vi "arm pid.vi"(2 "Setpoint":dbl, 3 "Autotune?":bool) -> (0 "Output":dbl)   [LabVIEW 2013]
uses:
  typedefs/fg_typedef.ctl
  typedefs/DevRef Type.ctl
  <vilib>/addons/control/pid/pid.llb/PID (DBL).vi
  <vilib>/addons/control/pid/NI_PID_autopid.lvlib
  <vilib>/addons/control/pid/NI_PID_pid.lvlib
panel:
  in  "autotuning parameters":T1={"controller type"=1, "relay cycles"=3, "relay amplitude"=1.0, "control specification"=2, "PV noise level"=0.1} {"controller type" items=["PID", "PI", "P"]; "control specification" items=["normal", "fast", "slow"]}
  # "Things needing Tuning"
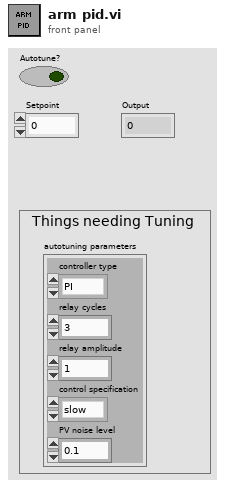
[diagram p1: front panel]
types:
  T1 = cluster{"controller type":u16, "relay cycles":i32, "relay amplitude":dbl, "control specification":u16, "PV noise level":dbl}
  T2 = cluster{"proportional gain (Kc)":dbl, "integral time (Ti, min)":dbl, "derivative time (Td, min)":dbl}
  T3 = typedef "DevRef Type.ctl" = enum16{"Shooter Solenoid", "Latch Solenoid", "Right Up Sensor", "Right Down Sensor", "Hold Sensor", "2 Ball Switch", "Arm Encoder"}
  T4 = typedef "fg_typedef.ctl" = enum16{"Get", "Set"}
  T5 = typedef "subStates.ctl" = enum16{"null", "wait", "driver control", "auto", "manual override", "hold position", "rotate", "pickup", "pass", "recover pass", "load", "goto shoot", "shoot high goal", "shoot low goal", "cancel arm", "cancel shooter", "end", "test"}
  T6 = typedef "WPI_EncoderDevRef.ctl" = cluster{"DevStatus":errorcluster, "EncoderIndex":T7, "CounterIndex":T8, "DistancePerCount":dbl, "Decoding Type":T9}
  T7 = typedef "FPGA_EncoderIdx.ctl" = enum8{"Enc 0", "Enc 1", "Enc 2", "Enc 3", "Invalid"}
  T8 = typedef "FPGA_CounterCtrSystemIndex.ctl" = enum8{"Ctr 0", "Ctr 1", "Ctr 2", "Ctr 3", "Ctr 4", "Ctr 5", "Ctr 6", "Ctr 7", "Invalid"}
  T9 = typedef "WPI_EncoderType.ctl" = enum16{"1x", "2x", "4x"}
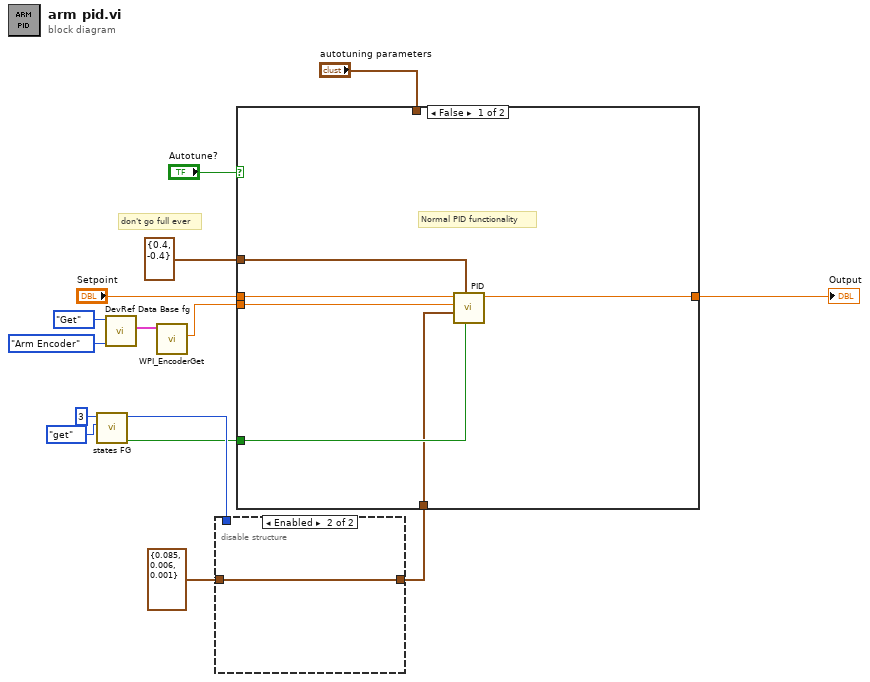
[diagram p0: block diagram]
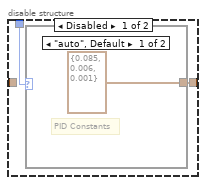
[diagram p2: hidden frame]
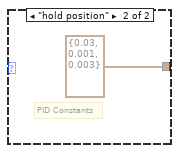
[diagram p3: hidden frame]
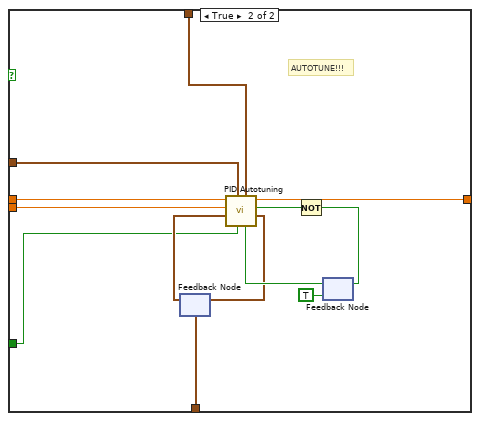
[diagram p4: hidden frame]
diagram:
  # "don't go full ever"
  n1 = call "states FG.vi"("menu (get)"=enum16{"set", "get"}."get", "Loop ID"=3) -> ("first call?"=w2:bool, "subState out"=w3:T5)  [unwired: 6 in, 2 out]
  n2 = call "DevRef Data Base fg.vi"("DevRef to Get"=DevRef_Type."Arm Encoder", "Menu"=fg_typedef."Get") -> ("Selected Encoder"=w7:T6)  [unwired: 2 in, 5 out]
  n3 = call <vilib>:"WPI_EncoderGet.vi"("EncoderDevRef"=w7) -> ("Distance"=w13:dbl)  [unwired: 5 in, 5 out]
  n4 = disable-structure shown="Enabled" {
    disable-tunnel: [w17 w20] -> w10
    disable-tunnel: w3 -> [w16 _]
    disable-tunnel: T2 {"proportional gain (Kc)"=0.085, "integral time (Ti, min)"=0.006, "derivative time (Td, min)"=0.001} ("PID gains") -> [_ w20]
    frame Disabled {
      n5 = case shown="\"auto\", Default" w16 {
        tunnel: [T2 {"proportional gain (Kc)"=0.085, "integral time (Ti, min)"=0.006, "derivative time (Td, min)"=0.001} ("PID gains") T2 {"proportional gain (Kc)"=0.03, "integral time (Ti, min)"=0.001, "derivative time (Td, min)"=0.003} ("Hold Position PID gains")] -> w17
        frame "auto", Default {
          # "PID Constants"
        }
        frame "hold position" {
          # "PID Constants"
        }
      }
    }
    frame Enabled {
    }
  }
  n6 = case shown="False" "Autotune?" {
    tunnel: "Setpoint" -> [w26 w39]
    tunnel: [w25 w38] -> w14
    tunnel: w13 -> [w23 w31]
    tunnel: w2 -> [w24 w30]
    tunnel: w10 -> [w22 w29]
    tunnel: cluster{"output high":dbl, "output low":dbl} {"output high"=0.4, "output low"=-0.4} ("output range") -> [w21 w28]
    tunnel: "autotuning parameters" -> [_ w27]
    frame False {
      # "Normal PID functionality"
      n7 = call-poly <vilib>:"PID.vi"("reinitialize? (F)"=w24, "output range"=w21, "PID gains"=w22, "process variable"=w23, "setpoint"=w26) -> ("output"=w25:dbl)  [unwired: 5 in, 1 out]
    }
    frame True {
      # "AUTOTUNE!!!"
      n8 = feedback #1(w29) -> (w32:T2)
      n9 = feedback #2(TRUE) -> (w35:bool)
      n10 = call <vilib>:"PID Autotuning.vi"("autotune? (F)"=w35, "autotuning parameters"=w27, "reinitialize? (F)"=w30, "output range"=w28, "PID gains"=w32, "process variable"=w31, "setpoint"=w39) -> ("PID gains out"=w33:T2, "tuning completed?"=w37:bool, "output"=w38:dbl)  [unwired: 1 in, 1 out]
      n11 = feedback-in #1(w33) -> ()
      n12 = Not(x=w37) -> (.not. x?=w36:bool)
      n13 = feedback-in #2(w36) -> ()
    }
  }
  "Output" <- w14
